vi "__CONST_INITIAL_ROOMS_STRING.vi"() -> (3 "inital rooms text":string caption="<JSON>Object")   [LabVIEW 2020, in "Room-API.lvclass"]
uses:
  Room-API.lvclass
  <vilib>/JDP Science/JSONtext/support/Format JSON Object.vi
  <vilib>/JDP Science/JSONtext/JSONtext.lvlib
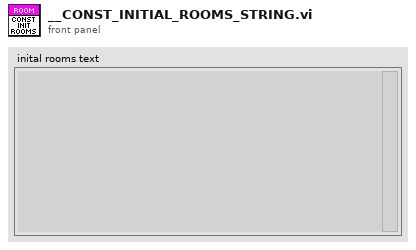
[diagram p1: front panel]
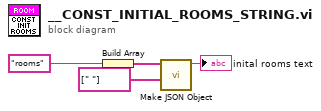
[diagram p0: block diagram]
diagram:
  n1 = Build Array("rooms") -> (w4:string[])
  n2 = call <vilib>:"Make JSON Object.vi"("JSON Items"=string[] [" "], "Item Names"=w4) -> ("<JSON>"=→"inital rooms text":string)  [unwired: 8 in, 1 out]
